vi "Init Msg Default.vi"() -> (2 "Msg":refnum<class "Msg.lvclass">)   [LabVIEW 2025, in "jettl.lvlib" / "Stopped jettl Msg.lvlib" / "Stopped Msg.lvlib"]
uses:
  Stopped Msg.lvlib
  Msg/Msg.lvclass
  Stopped Msg/Stopped Msg.lvclass
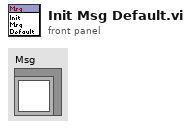
[diagram p1: front panel]
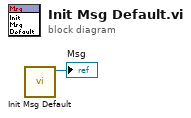
[diagram p0: block diagram]
diagram:
  n1 = call "Init Msg Default.vi"() -> ("Stopped Msg out"=→"Msg":refnum<class "Stopped Msg.lvclass">)  [unwired: 11 in]
